vi "TEST_CheckLevel.vi"() -> ()   [LabVIEW 2024]
doc: "This VI is used to test the Spec LUT (Look Up Table) Select ChA!ChB and Drain!Fill\nShould produce the spec index for the level entered.\nNote: Meausre shows the value whre Measure R is enabled."
uses:
  Control Definitions/Def FullCfg.ctl
  Control Definitions/Def BenchCfg.ctl
  Control Definitions/Def PumpCtlRefs.ctl
  Control Definitions/Def_PumpSpeed.ctl
  Control Definitions/Def Bench Status.ctl
  Control Definitions/Def_LevelSwitched.ctl
  Control Definitions/Def Spec RNG.ctl
  Control Definitions/Ded LUT_Status.ctl
  Control Definitions/Def Results2.ctl
panel:
  out "Results out":T1=[[{"Fill"=0.0, "Drain"=0.0, "Status"=0, "Resistor"=0.0}, {"Fill"=0.0, "Drain"=0.0, "Status"=0, "Resistor"=0.0}], [{"Fill"=0.0, "Drain"=0.0, "Status"=8, "Resistor"=0.0}, {"Fill"=0.0, "Drain"=0.0, "Status"=0, "Resistor"=0.0}], [{"Fill"=0.0, "Drain"=0.0, "Status"=0, "Resistor"=0.0}, {"Fill"=0.0, "Drain"=0.0, "Status"=0, "Resistor"=0.0}], [{"Fill"=0.0, "Drain"=0.0, "Status"=0, "Resistor"=0.0}, {"Fill"=0.0, "Drain"=0.0, "Status"=0, "Resistor"=0.0}], [{"Fill"=0.0, "Drain"=0.0, "Status"=0, "Resistor"=0.0}, {"Fill"=0.0, "Drain"=0.0, "Status"=0, "Resistor"=0.0}], [{"Fill"=0.0, "Drain"=0.0, "Status"=0, "Resistor"=0.0}, {"Fill"=0.0, "Drain"=0.0, "Status"=0, "Resistor"=0.0}], [{"Fill"=0.0, "Drain"=0.0, "Status"=0, "Resistor"=0.0}, {"Fill"=0.0, "Drain"=0.0, "Status"=0, "Resistor"=0.0}], [{"Fill"=0.0, "Drain"=0.0, "Status"=0, "Resistor"=0.0}, {"Fill"=0.0, "Drain"=0.0, "Status"=0, "Resistor"=0.0}], [{"Fill"=0.0, "Drain"=0.0, "Status"=0, "Resistor"=0.0}, {"Fill"=0.0, "Drain"=0.0, "Status"=0, "Resistor"=0.0}], [{"Fill"=0.0, "Drain"=0.0, "Status"=0, "Resistor"=0.0}, {"Fill"=0.0, "Drain"=0.0, "Status"=0, "Resistor"=0.0}], [{"Fill"=0.0, "Drain"=0.0, "Status"=0, "Resistor"=0.0}, {"Fill"=0.0, "Drain"=0.0, "Status"=0, "Resistor"=0.0}]] {"Resistor" format="%.1f"; "Drain" format="%.3f"; "Fill" format="%.3f"}
  out "element":T2
  out "Level Out":T4={"Switched"=FALSE, "Level OUt"=8.030499999999925}
  in  "Inputs":cluster{" Ohms":dbl, "Level OUt":dbl}={" Ohms"=101.0, "Level OUt"=8.030499999999925}
  in  "ChB!ChA":bool
  in  "Test Index":i32
  in  "Full Cfg 2":T5={"Bench Config"={"Name"="OLR001", {"Step Levels"=0.05, "Tolerance"=0.01, "Sample Rate"=0.05, "Resistor"=100.0, "M Level Cal"=1.0, "[B Level Cal"=0.0, "Max Fill Rate"=0.002, "Empty Inches"=8.0, "Full Inches"=2.6}}, "Test Value Table "=[[98.0, 102.0, 8.5, 8.5, 8.5, 8.5, 98.0, 102.0, 8.5, 8.5, 8.5, 8.5], [98.0, 102.0, 7.91, 8.01, 7.55, 7.65, 98.0, 102.0, 7.685, 7.785, 7.325, 7.425], [197.0, 203.0, 7.46, 7.56, 7.1, 7.2, 197.0, 203.0, 7.235, 7.335, 6.875, 6.975], [296.0, 304.0, 7.01, 7.11, 6.65, 6.75, 296.0, 304.0, 6.785, 6.885, 6.425, 6.525], [395.0, 405.0, 6.56, 6.66, 6.2, 6.3, 395.0, 405.0, 6.335, 6.435, 5.975, 6.075], [494.0, 506.0, 6.11, 6.21, 5.75, 5.85, 494.0, 506.0, 5.885, 5.985, 5.525, 5.625], [593.0, 607.0, 5.66, 5.76, 5.3, 5.4, 593.0, 607.0, 5.435, 5.535, 5.075, 5.175], [692.0, 708.0, 5.21, 5.31, 4.85, 4.95, 692.0, 708.0, 4.985, 5.085, 4.625, 4.725], [791.0, 809.0, 4.76, 4.86, 4.4, 4.5, 791.0, 809.0, 4.535, 4.635, 4.175, 4.275], [890.0, 910.0, 4.31, 4.41, 3.95, 4.05, 890.0, 910.0, 4.085, 4.185, 3.725, 3.825], [989.0, 1011.0, 3.86, 3.96, 3.5, 3.6, 989.0, 1011.0, 3.635, 3.735, 3.275, 3.375], [1088.0, 1112.0, 3.41, 3.51, 3.05, 3.15, 1088.0, 1112.0, 3.185, 3.285, 2.825, 2.925], [1088.0, 1112.0, 2.5, 2.5, 2.5, 2.5, 1088.0, 1112.0, 2.5, 2.5, 2.5, 2.5]], "Table Col Titles"=[["Aohm Lo", "Aohm Hi", "A Fill Lo", "A Fill Hi", "A Drain Lo", "A Drain Hi", "Bohm Lo", "Bohm Hi", "B Fill Lo", "B Fill Hi", "B Drain Lo", "B Drain Hi"]], "cluster"={"Fill "=refnum, "Drain"=refnum, "Level PV"=refnum, "Pump Speed"=refnum, "Run Test"=refnum, "Sim"=refnum, "Jog"=refnum, "Level SP"=refnum}, "Bench Status"={"Pump Status"=refnum, "Instrumnet\n Status"=refnum}}
  in  "stop":bool
  in  "Drain!Fill":bool
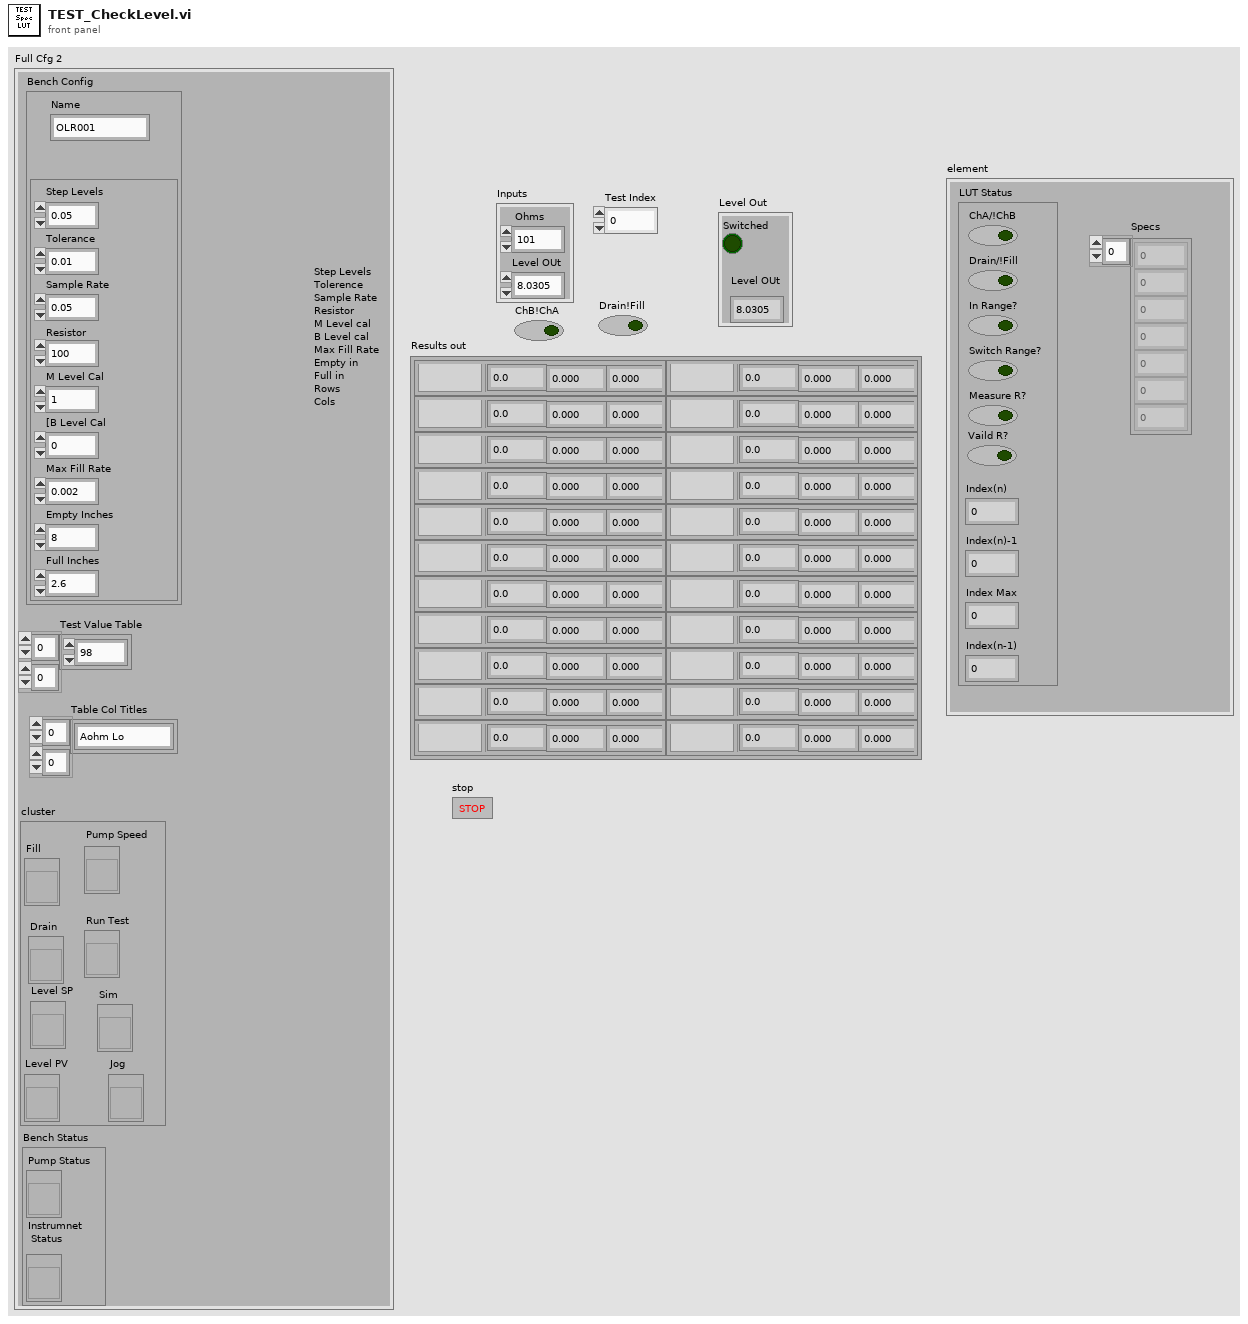
[diagram p1: front panel]
types:
  T1 = typedef "Def Results2.ctl" = cluster{"Fill":dbl, "Drain":dbl, "Status":i16, "Resistor":dbl}[][]
  T2 = typedef "Def Spec RNG.ctl" = cluster{"Specs":dbl[], "LUT Status":T3}
  T3 = typedef "Ded LUT_Status.ctl" = cluster{"ChA/!ChB":bool, "Drain/!Fill":bool, "In Range?":bool, "Switch Range?":bool, "Measure R?":bool, "Vaild R?":bool, "Index(n)":i32, "Index(n)-1":i32, "Index Max":i32, "Index(n-1)":i32}
  T4 = typedef "Def_LevelSwitched.ctl" = cluster{"Switched":bool, "Level OUt":dbl}
  T5 = typedef "Def FullCfg.ctl" = cluster{"Bench Config":T6, "Test Value Table ":dbl[][], "Table Col Titles":string[][], "cluster":T7, "Bench Status":T8}
  T6 = typedef "Def BenchCfg.ctl" = cluster{"Name":string, cluster{"Step Levels":dbl, "Tolerance":dbl, "Sample Rate":dbl, "Resistor":dbl, "M Level Cal":dbl, "[B Level Cal":dbl, "Max Fill Rate":dbl, "Empty Inches":dbl, "Full Inches":dbl}}
  T7 = typedef "Def PumpCtlRefs.ctl" = cluster{"Fill ":refnum<vi>, "Drain":refnum<vi>, "Level PV":refnum<vi>, "Pump Speed":refnum<vi>, "Run Test":refnum<vi>, "Sim":refnum<vi>, "Jog":refnum<vi>, "Level SP":refnum<vi>}
  T8 = typedef "Def Bench Status.ctl" = cluster{"Pump Status":refnum<vi>, "Instrumnet\n Status":refnum<vi>}
  T9 = cluster{"Spec RNG Out":T2[], "cluster":T7, "TEST State Out":u16, "Index":i32, "X>Pos":bool}
  T10 = cluster{"Fill":dbl, "Drain":dbl, "Status":i16, "Resistor":dbl}[]
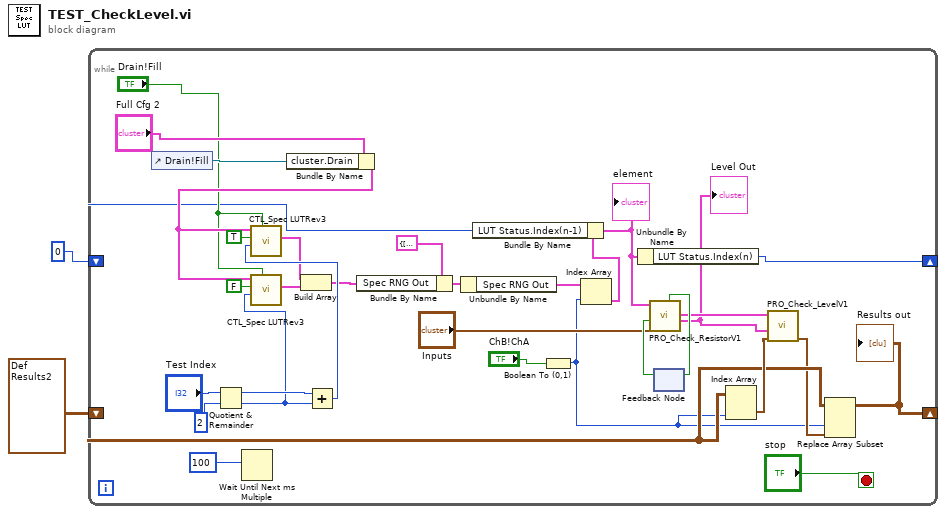
[diagram p0: block diagram]
diagram:
  n1 = while {
    shift-right: [w13] -> _
    shift-left: 0 ("Index(n)") -> [w10]
    shift-right: [w5] -> _
    shift-left: T1 [[{"Fill"=0.0, "Drain"=0.0, "Status"=0, "Resistor"=0.0}, {"Fill"=0.0, "Drain"=0.0, "Status"=0, "Resistor"=0.0}], [{"Fill"=0.0, "Drain"=0.0, "Status"=8, "Resistor"=0.0}, {"Fill"=0.0, "Drain"=0.0, "Status"=0, "Resistor"=0.0}], [{"Fill"=0.0, "Drain"=0.0, "Status"=0, "Resistor"=0.0}, {"Fill"=0.0, "Drain"=0.0, "Status"=0, "Resistor"=0.0}], [{"Fill"=0.0, "Drain"=0.0, "Status"=0, "Resistor"=0.0}, {"Fill"=0.0, "Drain"=0.0, "Status"=0, "Resistor"=0.0}], [{"Fill"=0.0, "Drain"=0.0, "Status"=0, "Resistor"=0.0}, {"Fill"=0.0, "Drain"=0.0, "Status"=0, "Resistor"=0.0}], [{"Fill"=0.0, "Drain"=0.0, "Status"=0, "Resistor"=0.0}, {"Fill"=0.0, "Drain"=0.0, "Status"=0, "Resistor"=0.0}], [{"Fill"=0.0, "Drain"=0.0, "Status"=0, "Resistor"=0.0}, {"Fill"=0.0, "Drain"=0.0, "Status"=0, "Resistor"=0.0}], [{"Fill"=0.0, "Drain"=0.0, "Status"=0, "Resistor"=0.0}, {"Fill"=0.0, "Drain"=0.0, "Status"=0, "Resistor"=0.0}], [{"Fill"=0.0, "Drain"=0.0, "Status"=0, "Resistor"=0.0}, {"Fill"=0.0, "Drain"=0.0, "Status"=0, "Resistor"=0.0}], [{"Fill"=0.0, "Drain"=0.0, "Status"=0, "Resistor"=0.0}, {"Fill"=0.0, "Drain"=0.0, "Status"=0, "Resistor"=0.0}], [{"Fill"=0.0, "Drain"=0.0, "Status"=0, "Resistor"=0.0}, {"Fill"=0.0, "Drain"=0.0, "Status"=0, "Resistor"=0.0}]] ("Results out") -> [w7]
    stop <- "stop" stop-if-true
    n2 = control-ref of="Drain!Fill"() -> (w36:refnum<vi>)
    n3 = Quotient & Remainder(x="Test Index", y=2) -> (x-y*floor(x/y)=w31:i32, floor(x/y)=w25:i32)
    n4 = Wait Until Next ms Multiple(millisecond multiple=u32 100) -> ()  [unwired: 1 out]
    n5 = Bundle By Name(cluster="Full Cfg 2", "cluster.Drain"=w36) -> (w24:T5)
    n6 = call "CTL_Spec LUTRev3.vi"("Drain!Fill"="Drain!Fill", "Index"=w25, "ChA/!ChB"=FALSE, "Full Cfg"=w24) -> ("Spec Range Out"=w26:T2)  [unwired: 4 in, 3 out]
    n7 = Add(x=w31, y=w25) -> (x+y=w28:i32)
    n8 = call "CTL_Spec LUTRev3.vi"("Drain!Fill"="Drain!Fill", "Index"=w28, "ChA/!ChB"=TRUE, "Full Cfg"=w24) -> ("Spec Range Out"=w27:T2)  [unwired: 4 in, 3 out]
    n9 = Build Array(w27, w26) -> (w20:T2[])
    n10 = Bundle By Name(cluster=T9 {"Spec RNG Out"=[], "cluster"={"Fill "=refnum, "Drain"=refnum, "Level PV"=refnum, "Pump Speed"=refnum, "Run Test"=refnum, "Sim"=refnum, "Jog"=refnum, "Level SP"=refnum}, "TEST State Out"=0, "Index"=0, "X>Pos"=FALSE}, "Spec RNG Out"=w20) -> (w19:T9)
    n11 = Unbundle By Name(w19) -> ("Spec RNG Out"=w18:T2[])
    n12 = Boolean To (0,1)(Boolean="ChB!ChA") -> (0, 1=w3:i16)
    n13 = Index Array(array=w18, index=w3) -> (element=w12:T2)
    n14 = Bundle By Name(cluster=w12, "LUT Status.Index(n-1)"=w10) -> (w11:T2)
    "element" <- w11
    n15 = Unbundle By Name(w11) -> ("LUT Status.Index(n)"=w13:i32)
    n16 = feedback #1() -> (w15:bool)  [unwired: 1 in]
    n17 = call "PRO_Check_ResistorV1.vi"("Switched In"=w15, "Inputs"="Inputs", "ChA Spec RNG In"=w11) -> ("Level Out"=w4:T4, "ChA Spec RNG Out"=w9:T2, "Switched Out"=w16:bool)  [unwired: 4 in, 2 out]
    "Level Out" <- w4
    n18 = feedback-in #1(w16) -> ()
    n19 = Index Array(array=w7, index (col)=w3) -> (element=w8:T10)  [unwired: 1 in]
    n20 = call "PRO_Check_LevelV1.vi"("Results In"=w8, "Level In"=w4, "ChA Spec RNG In"=w9) -> ("Results Out"=w6:T10)  [unwired: 5 in, 3 out]
    n21 = Replace Array Subset(array=w7, new element=w6, index (col)=w3) -> (w5:T1)  [unwired: 1 in]
    "Results out" <- w5
  }
